vi "maquina estados.vi"() -> ()   [LabVIEW 2014]
uses:
  Control 4.ctl
panel:
  in  "# Maximo":dbl
  in  "Numeric":dbl
  in  "stop":bool
  in  "Decremento":bool
  in  "Incremento":bool
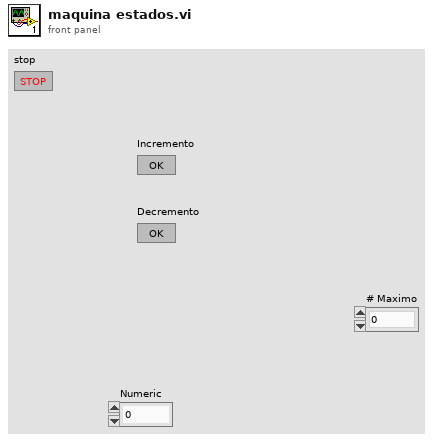
[diagram p1: front panel]
types:
  T1 = typedef "Control 4.ctl" = enum16{"S0", "S1", "S2", "S3", "S4"}
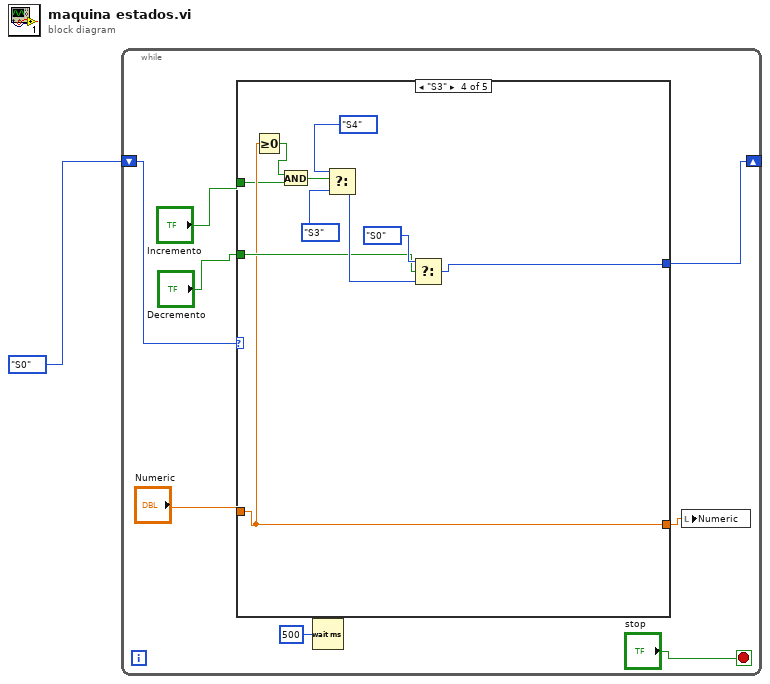
[diagram p0: block diagram]
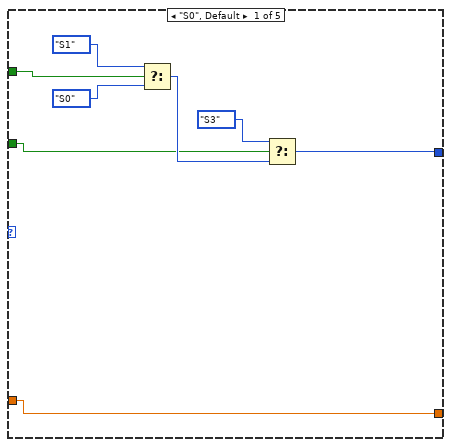
[diagram p2: hidden frame]
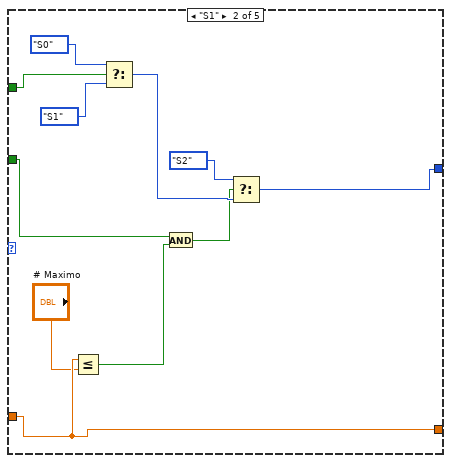
[diagram p3: hidden frame]
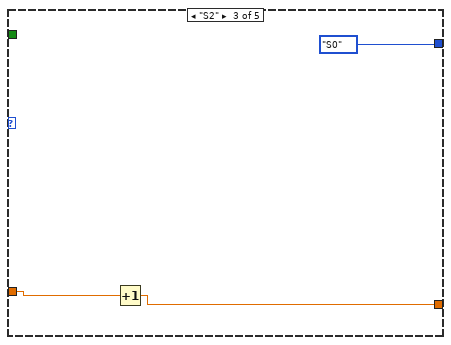
[diagram p4: hidden frame]
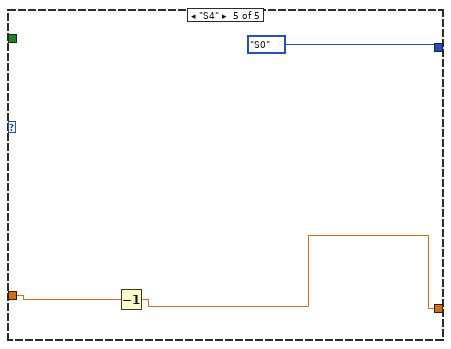
[diagram p5: hidden frame]
diagram:
  n1 = while {
    shift-right: [w9] -> _
    shift-left: Control_4."S0" -> [w5]
    stop <- "stop" stop-if-true
    n2 = case shown="\"S3\"" w5 {
      tunnel: [w13 w23 Control_4."S0" w37 Control_4."S0"] -> w9
      tunnel: "Incremento" -> [w12 w28 _ w32 _]
      tunnel: "Decremento" -> [w11 w22 _ w36 _]
      tunnel: "Numeric" -> [w10 w20 w30 w35 w43]
      tunnel: [w10 w20 w29 w35 w42] -> w3
      frame "S0", Default {
        n3 = Select(t=Control_4."S1", s=w12, f=Control_4."S0") -> (s? t:f=w17:T1)
        n4 = Select(t=Control_4."S3", s=w11, f=w17) -> (s? t:f=w13:T1)
      }
      frame "S1" {
        n5 = Less Or Equal?(x=w20, y="# Maximo") -> (x <= y?=w18:bool)
        n6 = Select(t=Control_4."S0", s=w28, f=Control_4."S1") -> (s? t:f=w25:T1)
        n7 = And(x=w22, y=w18) -> (x .and. y?=w21:bool)
        n8 = Select(t=Control_4."S2", s=w21, f=w25) -> (s? t:f=w23:T1)
      }
      frame "S2" {
        n9 = Increment(x=w30) -> (x+1=w29:dbl)
      }
      frame "S3" {
        n10 = Greater Or Equal To 0?(x=w35) -> (x >= 0?=w33:bool)
        n11 = And(x=w33, y=w32) -> (x .and. y?=w34:bool)
        n12 = Select(t=Control_4."S4", s=w34, f=Control_4."S3") -> (s? t:f=w38:T1)
        n13 = Select(t=Control_4."S0", s=w36, f=w38) -> (s? t:f=w37:T1)
      }
      frame "S4" {
        n14 = Decrement(x=w43) -> (x-1=w42:dbl)
      }
    }
    n15 = Wait (ms)(milliseconds to wait=u32 500) -> ()  [unwired: 1 out]
    n16 = local write "Numeric"(w3) -> ()
  }
